vi "Cowl_Globals.vi"() -> ()   [LabVIEW 2019]
uses:
  Cowl_Cluster.ctl
  Cowl_States.ctl
  Utility VIs/Basic_Motor_Modes.ctl
panel:
  out "Cowl_Absolute_Position (Degrees)":dbl
  out "Cowl_Goal":dbl
  in  "Basic_Motor_Mode":T1
  out "Cowl_Output":dbl
  in  "Cowl_Set_Notifier":refnum<notifier>
  in  "Cowl_Execute_Notifier":refnum<notifier>
  in  "Cowl_Execute_Ref":string="Cowl_Execute_Ref"
  in  "Cowl_Set_Ref":string="Cowl_Set_Ref"
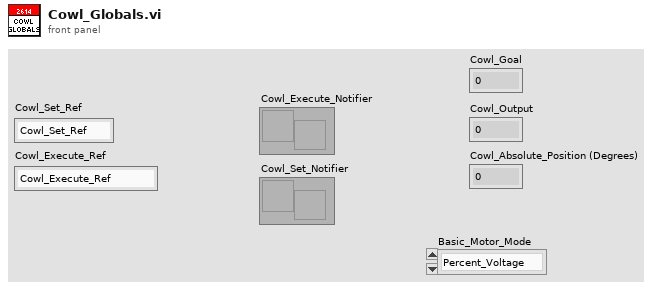
[diagram p1: front panel]
types:
  T1 = typedef "Basic_Motor_Modes.ctl" = enum16{"Percent_Voltage", "Speed_Control", "Position_Control", "Current"}
diagram:
